vi "Build_waveform.vi"(8 "error in (no error)":errorcluster, 11 "build_waveform in":refnum<class "build_waveform.lvclass">) -> (0 "error out":errorcluster, 2 "Array":dbl[](array[numeric]), 3 "build_waveform out":refnum<class "build_waveform.lvclass">)   [LabVIEW 2015, in "build_waveform.lvclass"]
uses:
  build_waveform.lvclass
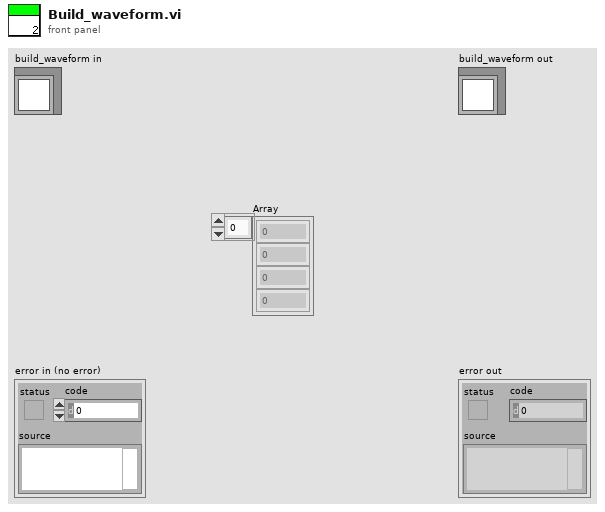
[diagram p1: front panel]
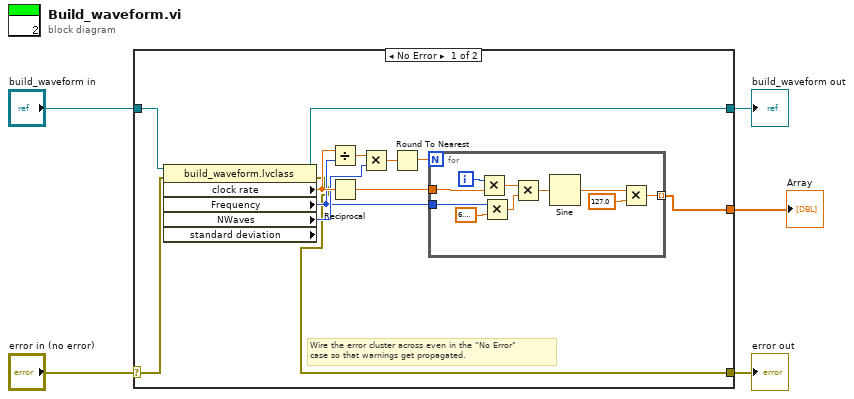
[diagram p0: block diagram]
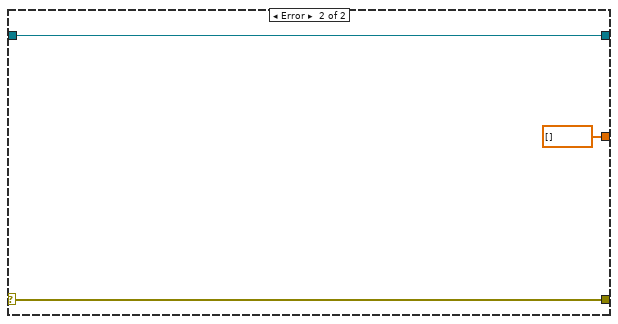
[diagram p2: hidden frame]
diagram:
  n1 = case shown="No Error" "error in (no error)" {
    selector: "error in (no error)" -> [w8 w30]
    tunnel: [w7 w30] -> w4
    tunnel: [w9 w29] -> w2
    tunnel: "build_waveform in" -> [w10 w29]
    tunnel: [w6 dbl[] []] -> w1
    frame No Error {
      # "Wire the error cluster across even in the \"No Error\"\ncase so that warnings get propagated."
      n2 = property class="build_waveform.lvclass" props=["clock rate", "Frequency", "NWaves", "standard deviation"](reference=w10, error in=w8) -> (reference out=w9:refnum<class "build_waveform.lvclass">, error out=w7:errorcluster, "clock rate"=w17:dbl, "Frequency"=w12:i32, "NWaves"=w16:i32)  [unwired: 1 out]
      n3 = Divide(x=w17, y=w12) -> (x/y=w15:dbl)
      n4 = Reciprocal(x=w17) -> (1/x=w11:dbl)
      n5 = Multiply(x=w15, y=w16) -> (x*y=w14:dbl)
      n6 = Round To Nearest(number=w14) -> (nearest integer value=w13:dbl)
      n7 = for {
        N: w13 -> [_]
        tunnel: [w21] -> w6 mode=indexing
        tunnel: w12 -> [w18]
        tunnel: w11 -> [w19]
        i -> [w20]
        n8 = Multiply(x=w20, y=w19) -> (x*y=w23:dbl)
        n9 = Multiply(x=w18, y=6.283185307179586) -> (x*y=w24:dbl)
        n10 = Multiply(x=w23, y=w24) -> (x*y=w26:dbl)
        n11 = Sine(x=w26) -> (sin(x)=w22:dbl)
        n12 = Multiply(x=w22, y=127.0) -> (x*y=w21:dbl)
      }
    }
    frame Error {
    }
  }
  "error out" <- w4
  "build_waveform out" <- w2
  "Array" <- w1
